vi "Execute Python Optimization (Off-Grid).vi"(6 "Results Queue":refnum<queue>, 8 "error in":errorcluster, 11 "Off-Grid in":refnum<class "Off-Grid.lvclass">) -> (0 "error out":errorcluster, 3 "Off-Grid out":refnum<class "Off-Grid.lvclass">)   [LabVIEW 2018, in "Off-Grid Actor.lvlib" / "Off-Grid.lvclass"]
uses:
  Off-Grid.lvclass
  C:/Users/Administrator/Desktop/LabVIEW EMS/Optimization/Generic Optimization Actor/Generic Optimization/Generic Optimization.lvclass
  Generic Optimization Actor/Generic Optimization/Controls/Grid State for Optimization.ctl
  Global Variables/Global Variables.vi
  Generic Optimization Actor/Generic Optimization/Generic Optimization.lvclass
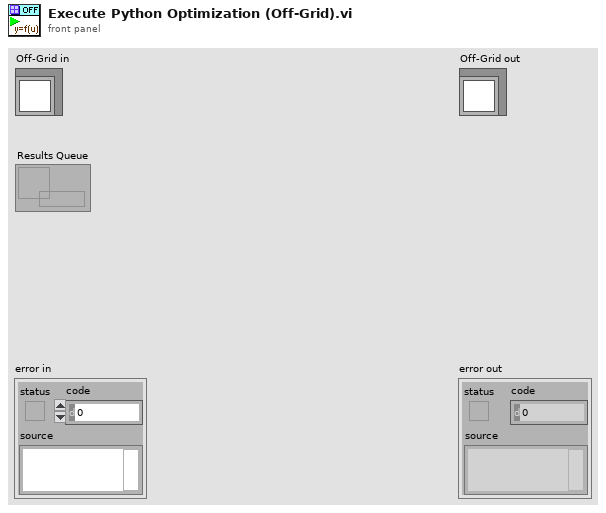
[diagram p1: front panel]
types:
  T1 = typedef "Generic Optimization Actor.lvlib/Generic Optimization.lvclass/Grid State for Optimization.ctl" = enum16{"Invalid", "On-Grid", "Off-Grid", "Island", "Resynch", "Blackstart", "Networked"}
  T2 = typedef "Optimization Type Selector.ctl" = enum16{"Invalid", "Single Phase", "Volttron"}
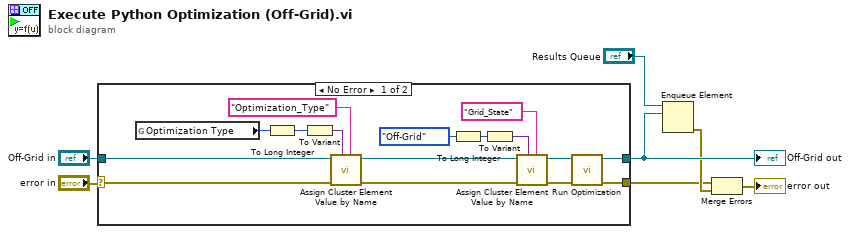
[diagram p0: block diagram]
diagram:
  n1 = case shown="No Error" "error in" {
    selector: "error in" -> [w14 w25]
    tunnel: [w8 w25] -> w2
    tunnel: [w9 w24] -> w4
    tunnel: "Off-Grid in" -> [w12 w24]
    frame No Error {
      n2 = global read "Global Variables.vi" "Optimization Type"() -> (w18:T2)
      n3 = To Long Integer(number=w18) -> (32bit integer=w19:i32)
      n4 = To Variant(anything=w19) -> (Variant=w17:variant)
      n5 = call "Assign Cluster Element Value by Name.vi"("Element Name"="Optimization_Type" ("Keyword Name"), "Value"=w17, "error in"=w14, "Generic Optimization"=w12) -> ("error out"=w15:errorcluster, "Generic Optimization out"=w13:refnum<class "Off-Grid.lvclass">)  [unwired: 6 in]
      n6 = To Long Integer(number=Grid_State_for_Optimization."Off-Grid") -> (32bit integer=w20:i32)
      n7 = To Variant(anything=w20) -> (Variant=w22:variant)
      n8 = call "Assign Cluster Element Value by Name.vi"("Element Name"="Grid_State" ("Keyword Name"), "Value"=w22, "error in"=w15, "Generic Optimization"=w13) -> ("error out"=w10:errorcluster, "Generic Optimization out"=w11:refnum<class "Off-Grid.lvclass">)  [unwired: 6 in]
      n9 = call "Run Optimization.vi"("error in"=w10, "Generic Optimization"=w11) -> ("error out"=w8:errorcluster, "Generic Optimization out"=w9:refnum<class "Off-Grid.lvclass">)  [unwired: 8 in]
    }
    frame Error {
    }
  }
  "Off-Grid out" <- w4
  n10 = Enqueue Element(queue="Results Queue", element=w4) -> (error out=w3:errorcluster)  [unwired: 2 in, 2 out]
  n11 = Merge Errors(w2, w3) -> (→"error out":errorcluster)
